vi "Page_Source_Can_Add_to_Top.vi"(6 "Project Refnum":refnum<vi>, 8 "error in (no error)":errorcluster, 10 "AB_Source in":refnum<class "AB_Source.lvclass">, 11 "AB_Targetfile in":refnum<class "AB_Targetfile.lvclass">) -> (0 "error out":errorcluster, 1 "message":string, 2 "canAddToTop":bool, 3 "AB_Targetfile out":refnum<class "AB_Targetfile.lvclass">)   [LabVIEW 2020, in "AB_Targetfile.lvclass"]
uses:
  <vilib>/AppBuilder/AB_Classes/TargetFile/AB_Targetfile.lvclass
  <vilib>/AppBuilder/AB_Classes/Source/AB_Source.lvclass
  <resource>/Framework/Providers/Common/provcom_StringGlobals.vi
  <vilib>/AppBuilder/AB_Classes/TargetFile/AB_Targetfile.lvclass/AB_Targetfile.ctl
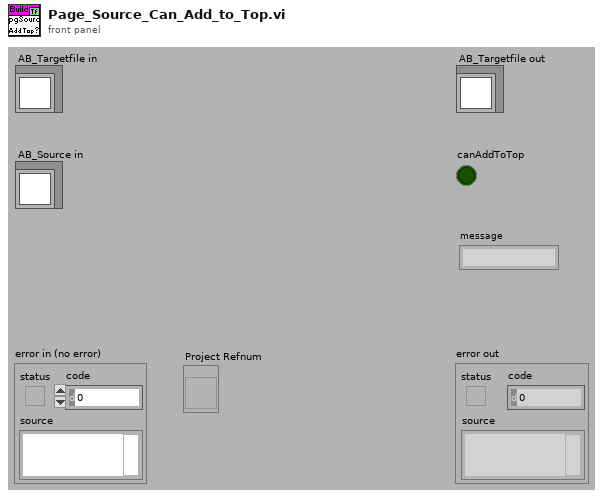
[diagram p1: front panel]
types:
  T1 = typedef "AB_Source.ctl" = cluster{"path":path, "itemID":string, "parentIndex":i32, "sourceInclusion":T2, "destinationIndex":i32, "properties":T3[], "newName":string, "lvfile":bool, "valid":bool, "eng_inBuild":bool, "eng_isNonVILink":bool, "Amalgamation":bool, "Amalgamation Piece":bool, "eng_delimitedName":string, "preventRename":bool}
  T2 = typedef "AB_Source_Inclusion.ctl" = enum16{"IncludeIfReferenced", "Include", "Exclude", "TopLevel"}
  T3 = typedef "AB_Source_Properties.ctl" = cluster{"sourcePropertyType":T4, "value":variant}
  T4 = typedef "AB_Source_Property_Type.ctl" = enum16{"Remove block diagram", "Remove front panel", "Password", "Window has title bar", "Show menu bar", "Show vertical scroll bar", "Show horizontal scroll bar", "Show toolbar", "Show Abort button", "Show fp when called", "Window behavior", "Allow user to close window", "Window run-time position", "Run when opened", "Allow debugging", "Auto error handling", "Generate guard code", "Use stack variables", "Expression folding", "Integer only", "Inline subVI"}
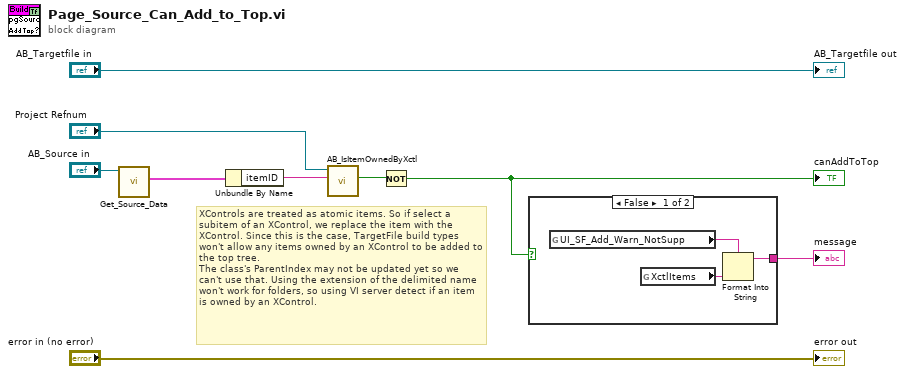
[diagram p0: block diagram]
diagram:
  # "XControls are treated as atomic items. So if select a subitem of an XControl, we replace the item with the XControl. Since this is the case, TargetFile build types won't allow any items owned by an XControl to be added to the top tree.\nThe class's ParentIndex may not be updated yet so we can't use that. Using the extension of the delimited name won't work for folders, so using VI server detect if an item is owned by an XControl."
  n1 = call <vilib>:"Get_Source_Data.vi"("Class in"="AB_Source in") -> ("data"=w8:T1)  [unwired: 8 in, 2 out]
  n2 = Unbundle By Name(w8) -> ("itemID"=w4:string)
  n3 = call <vilib>:"AB_IsItemOwnedByXctl.vi"("itemID"=w4, "Project Refnum"="Project Refnum") -> ("owned?"=w3:bool)  [unwired: 8 in, 1 out]
  n4 = Not(x=w3) -> (.not. x?=w2:bool)
  "canAddToTop" <- w2
  n5 = case shown="False" w2 {
    tunnel: [w10 _] -> w6
    frame False {
      n6 = global read "provcom_StringGlobals.vi" "UI_SF_Add_Warn_NotSupp"() -> (w12:string)
      n7 = global read "provcom_StringGlobals.vi" "XctlItems"() -> (w11:string)
      n8 = Format Into String(format string=w12, w11) -> (resulting string=w10:string)  [unwired: 2 in, 1 out]
    }
    frame True {
    }
  }
  "message" <- w6
  "error out" <- "error in (no error)"
  "AB_Targetfile out" <- "AB_Targetfile in"
